vi "DAQ Globals.vi"() -> ()   [LabVIEW 2020]
panel:
  out "Pinch Valve Disengage":refnum<k21>
  out "Pinch Valve Engage":refnum<k21>
  out "Cartridge Sensors":refnum<k21>
  out "Pressure Sensors":refnum<k21>
  in  "DAQ Rate":dbl=5000.0
  in  "DAQ Samples":i32=100
  # "DAQ Analog Outputs"
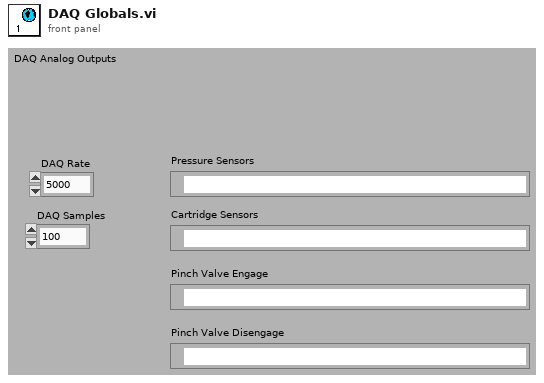
[diagram p1: front panel]
diagram:
